vi "Init Lift Motor With CVS File.vi"(2 "error in":errorcluster, 3 "Robot ID":string="981") -> (0 "error out":errorcluster)   [LabVIEW 2018]
panel:
  out "Lift Can Motor ID":u8
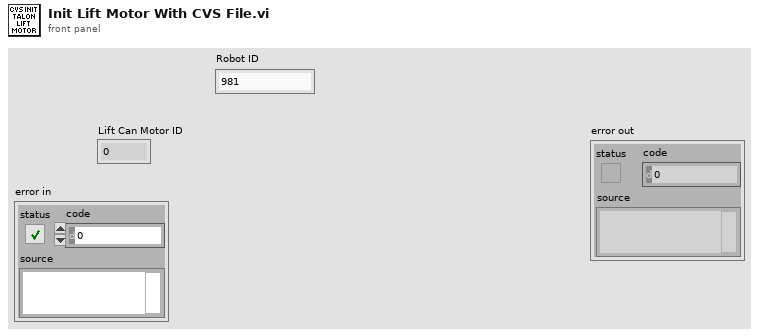
[diagram p1: front panel]
types:
  T1 = typedef "WPI_MotorControlDeviceRef.ctl" = cluster{"DeviceStatus":errorcluster, "Type":T2, "PWM":cluster{"PWM Channel":T3, "DeadBand":T4}, "CAN":cluster{"Device Number":u8, "SetOutput VI Ref":variant, "GetOutput VI Ref":variant, "Enable VI Ref":variant, "Disable VI Ref":variant, "Data":variant}, "Invert":bool, "DIO PWM":cluster{"PWM \"Enable\" Channel":T3, "DIOChannel":T5, "PWM Rate":dbl}}
  T2 = typedef "WPI_MotorControlType.ctl" = enum16{"PWM", "CAN", "DIO PWM"}
  T3 = typedef "FPGA_DIOPWMChannel.ctl" = enum8{"PWM 0", "PWM 1", "PWM 2", "PWM 3", "PWM 4", "PWM 5", "PWM 6", "PWM 7", "PWM 8", "PWM 9", "PWM MXP 0", "PWM MXP 1", "PWM MXP 2", "PWM MXP 3", "PWM MXP 4", "PWM MXP 5", "PWM MXP 6", "PWM MXP 7", "PWM MXP 8", "PWM MXP 9", "Invalid"}
  T4 = typedef "WPI_PWMDeadband.ctl" = cluster{"Name":string, "maxPositivePwm":i32, "minPositivePwm":i32, "centerPwm":i32, "maxNegativePwm":i32, "minNegativePwm":i32, "angularRange":u16}
  T5 = typedef "FPGA_DIOChannel.ctl" = enum8{"DIO 0", "DIO 1", "DIO 2", "DIO 3", "DIO 4", "DIO 5", "DIO 6", "DIO 7", "DIO 8", "DIO 9", "DIO MXP 0", "DIO MXP 1", "DIO MXP 2", "DIO MXP 3", "DIO MXP 4", "DIO MXP 5", "DIO MXP 6", "DIO MXP 7", "DIO MXP 8", "DIO MXP 9", "DIO MXP 10", "DIO MXP 11", "DIO MXP 12", "DIO MXP 13", "DIO MXP 14", "DIO MXP 15", "SPI Port CS1", "SPI Port CS2", "SPI Port CS3", "SPI Port MISO", "SPI Port MOSI", "Invalid"}
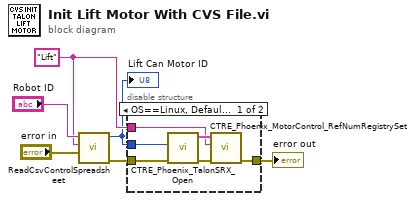
[diagram p0: block diagram]
diagram:
  w5 = "Lift" ("Motor ID")
  n1 = call "ReadCsvControlSpreadsheet.vi"("error in"="error in", "Motor ID"=w5, "Robot ID"="Robot ID") -> ("error out"=w4:errorcluster, "Can Bus ID"=w1:u8)  [unwired: 7 out]
  "Lift Can Motor ID" <- w1
  n2 = disable-structure shown="OS==Linux, Default" {
    disable-tunnel: w1 -> [w12 _]
    disable-tunnel: w5 -> [w10 _]
    disable-tunnel: w4 -> [w9 w13]
    disable-tunnel: [w7 w13] -> w3
    frame condition #0 (active) {
      n3 = call <vilib>:"CTRE_Phoenix_TalonSRX_Open.vi"("error in"=w9, "Device Number"=w12) -> ("error out"=w8:errorcluster, "CAN Talon SRX Ref"=w11:T1)  [unwired: 8 in]
      n4 = call <vilib>:"CTRE_Phoenix_MotorControl_RefNumRegistrySet.vi"("error in (no error)"=w8, "refnum name"=w10, "PhoenixMotorControlDevRef"=w11) -> ("error out"=w7:errorcluster)  [unwired: 7 in, 1 out]
    }
    frame condition #1 {
    }
  }
  "error out" <- w3
